vi "Read Channel URL list.vi"(8 "error in":errorcluster, 11 "Module Editor Node in":refnum<class "module editor node.lvclass">) -> (0 "error out":errorcluster, 2 "URLs":string[](array[string]), 3 "Module Editor Node out":refnum<class "module editor node.lvclass">)   [LabVIEW 2013, in "PL Framework Configuration Tool.lvlib" / "module editor node.lvclass"]
uses:
  module editor node.lvclass
  <vilib>/NI/Tag Bus/tag/tag descriptor.lvclass/tag descriptor.ctl
  <vilib>/NI/Tag Bus Module Framework/module configuration/TBM module configuration.lvclass
  <vilib>/NI/Tag Bus/tag/tag descriptor.lvclass
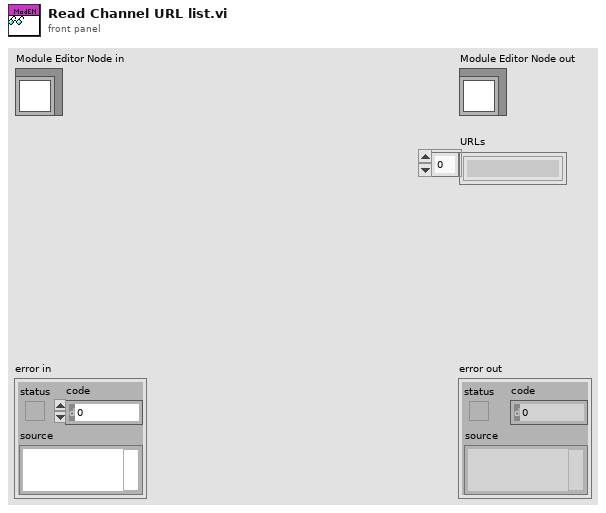
[diagram p1: front panel]
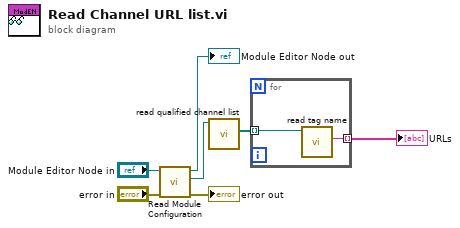
[diagram p0: block diagram]
diagram:
  n1 = call "Read Module Configuration.vi"("error in"="error in", "Module Editor Node in"="Module Editor Node in") -> ("error out"=→"error out":errorcluster, "module configuration"=w1:refnum<class "TBM module configuration.lvclass">, "Module Editor Node out"=→"Module Editor Node out":refnum<class "module editor node.lvclass">)  [unwired: 7 in]
  n2 = call <vilib>:"read qualified channel list.vi"("module configuration in"=w1) -> ("qualified channels"=w5:refnum<class "TBM channel.lvclass">[])  [unwired: 9 in, 1 out]
  n3 = for {
    tunnel: w5 -> [w9] mode=indexing
    tunnel: [w8] -> w4 mode=indexing
    n4 = call <vilib>:"read tag name.vi"("system tag in"=w9) -> ("name"=w8:string)  [unwired: 8 in, 2 out]
  }
  "URLs" <- w4
